vi "SeCrTs-Event logger.vi"(8 "error IO":errorcluster, 11 "?":T1) -> ()   [LabVIEW 2022 SP3]
uses:
  UI Message handler/Message Queue/All Message Queues.ctl
  UI Message handler/Message Queue/Message Cluster.ctl
  Controls/SeCrTs-Control error log.ctl
  UI Message handler/Message Queue/Message Queue.lvlib
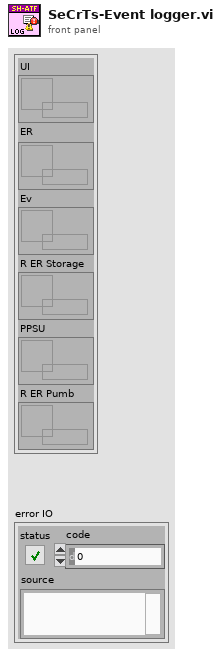
[diagram p1: front panel]
types:
  T1 = typedef "Message Queue.lvlib/All Message Queues.ctl" = cluster{"UI":refnum<queue>, "ER":refnum<queue>, "Ev":refnum<queue>, "R ER Storage":refnum<queue>, "PPSU":refnum<queue>, "R ER Pumb":refnum<queue>}
  T2 = typedef "SeCrTs-Control error log.ctl" = enum16{"Initialise", "Poll Event", "Logg Error", "Exit"}
  T3 = enum16{"open", "replace", "create", "open or create", "replace or create", "replace or create with confirmation"}
  T4 = typedef "SeCrTs-file folder ctl.ctl" = cluster{"Datalog path":path, "Configuration path":path, "Signal list path":path, "Sub vi's":path, "Authentication":path, "Sequence":path, "Event Log":path, "CS Error log":path, "RT Error Log":path}
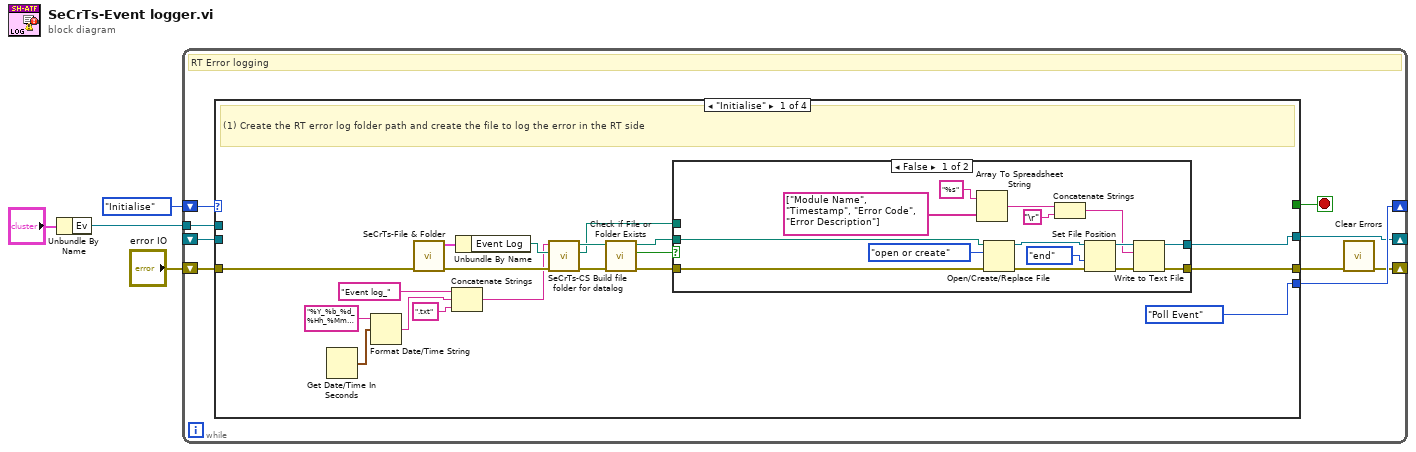
[diagram p0: block diagram]
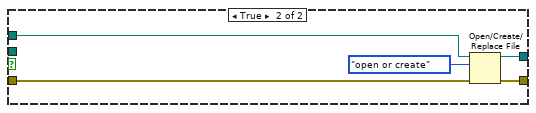
[diagram p2: hidden frame]
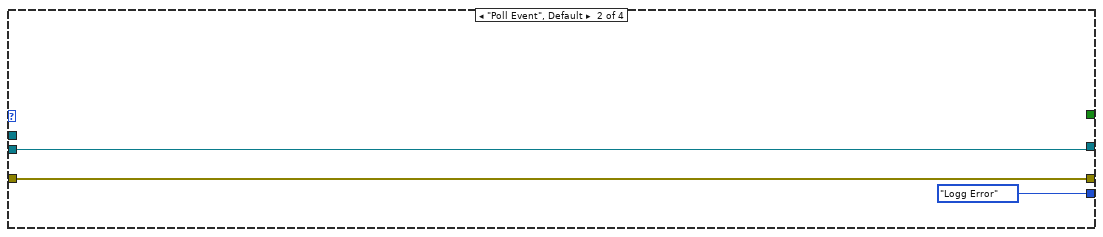
[diagram p3: hidden frame]
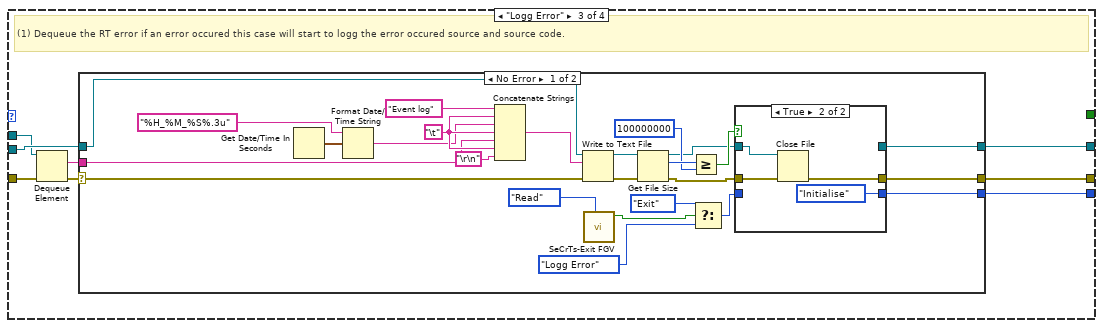
[diagram p4: hidden frame]
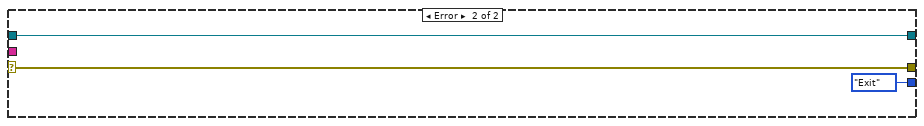
[diagram p6: hidden frame]
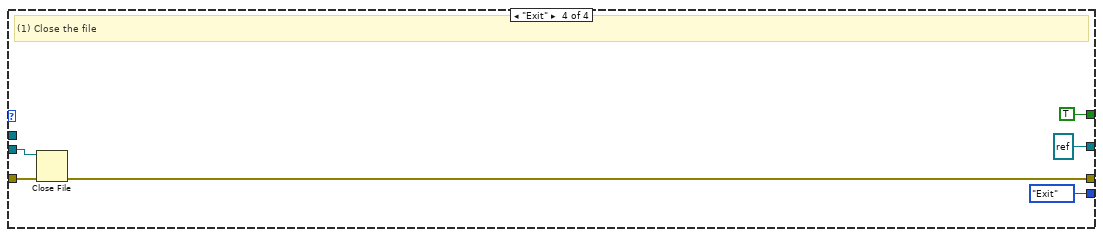
[diagram p7: hidden frame]
diagram:
  n1 = Unbundle By Name("?") -> ("Ev"=w1:refnum<queue>)
  n2 = while {
    shift-right: [w12] -> _
    shift-left: SeCrTs-Control_error_log."Initialise" -> [w13]
    shift-right: [w11] -> _
    shift-left: _ -> [w10]
    shift-right: [w5] -> _
    shift-left: "error IO" -> [w9]
    tunnel: w1 -> [w6]
    stop <- w7 stop-if-true
    # "RT Error logging"
    n3 = case shown="\"Initialise\"" w13 {
      tunnel: [SeCrTs-Control_error_log."Poll Event" SeCrTs-Control_error_log."Logg Error" w57 SeCrTs-Control_error_log."Exit"] -> w12
      tunnel: [w22 w55 w61 refnum<file> refnum ("refnum out")] -> w11
      tunnel: w10 -> [_ w55 w62 w102]
      tunnel: w9 -> [w19 w54 w59 w101]
      tunnel: [w20 w54 w60 w100] -> w8
      tunnel: [_ _ _ TRUE] -> w7
      tunnel: w6 -> [_ _ w56 _]
      frame "Initialise" {
        # "(1) Create the RT error log folder path and create the file to log the error in the RT side"
        n4 = Get Date/Time In Seconds() -> (seconds since 1Jan1904=w15:timestamp)
        n5 = Format Date/Time String(time format string (%c)="%Y_%b_%d_%Hh_%Mm_%Ssec", seconds (now)=w15) -> (date/time string=w14:string)  [unwired: 1 in]
        n6 = call "SeCrTs-File & Folder.vi"("error in (no error)"=w19) -> ("error out"=w31:errorcluster, "File Output"=w32:T4)  [unwired: 9 in]
        n7 = Concatenate Strings("Event log_" ("string"), w14, ".txt" ("string")) -> (w25:string)
        n8 = Unbundle By Name(w32) -> ("Event Log"=w30:path)
        n9 = call "SeCrTs-CS Build file folder for datalog.vi"("error in (no error)"=w31, "Base Path"=w30, "File Name"=w25) -> ("error out"=w28:errorcluster, "Result File path"=w17:path, "Result Folder path"=w29:path)  [unwired: 6 in]
        n10 = call <vilib>:"Check if File or Folder Exists.vi"("error in (no error)"=w28, "path"=w29) -> ("error out"=w21:errorcluster, "file or folder exists?"=w23:bool, "dup path"=w18:path)  [unwired: 7 in]
        n11 = case shown="False" w23 {
          tunnel: [w43 w51] -> w22
          tunnel: w21 -> [w46 w50]
          tunnel: [w42 w49] -> w20
          tunnel: w18 -> [w33 _]
          tunnel: w17 -> [_ w48]
          frame False {
            n12 = Array To Spreadsheet String(array=string[] ["Module Name", "Timestamp", "Error Code", "Error Description"], 3:"%s" ("format string")) -> (spreadsheet string=w37:string)  [unwired: 1 in]
            n13 = Open/Create/Replace File(file path (use dialog)=w33, error in=w46, operation (0:open)=T3."open or create") -> (refnum out=w45:refnum<file>, error out=w44:errorcluster)  [unwired: 3 in, 1 out]
            n14 = Concatenate Strings(w37, "\r") -> (w35:string)
            n15 = Set File Position(refnum=w45, from (0:start)=enum16{"start", "end", "current"}."end", error in=w44) -> (refnum out=w41:refnum<file>, error out=w40:errorcluster)  [unwired: 1 in]
            n16 = Write to Text File(file (use dialog)=w41, text=w35, error in=w40) -> (refnum out=w43:refnum<file>, error out=w42:errorcluster)  [unwired: 1 in, 1 out]
          }
          frame True {
            n17 = Open/Create/Replace File(file path (use dialog)=w48, error in=w50, operation (0:open)=T3."open or create") -> (refnum out=w51:refnum<file>, error out=w49:errorcluster)  [unwired: 3 in, 1 out]
          }
        }
      }
      frame "Poll Event", Default {
      }
      frame "Logg Error" {
        # "(1) Dequeue the RT error if an error occured this case will start to logg the error occured source and source code."
        n18 = Dequeue Element(queue=w56, error in (no error)=w59) -> (element=w63:string, error out=w58:errorcluster)  [unwired: 1 in, 2 out]
        n19 = case shown="No Error" w58 {
          selector: w58 -> [w83 w98]
          tunnel: w63 -> [w66 _]
          tunnel: w62 -> [w88 w97]
          tunnel: [w73 w97] -> w61
          tunnel: [w75 w98] -> w60
          tunnel: [w72 SeCrTs-Control_error_log."Exit"] -> w57
          frame No Error {
            w86 = "\t"
            n20 = Get Date/Time In Seconds() -> (seconds since 1Jan1904=w64:timestamp)
            n21 = Format Date/Time String(time format string (%c)="%H_%M_%S%.3u", seconds (now)=w64) -> (date/time string=w85:string)  [unwired: 1 in]
            n22 = Concatenate Strings("Event log" ("string"), w86, w85, w86, w66, w86, "\r\n") -> (w69:string)
            n23 = Write to Text File(file (use dialog)=w88, text=w69, error in=w83) -> (refnum out=w80:refnum<file>, error out=w81:errorcluster)  [unwired: 1 in, 1 out]
            n24 = call "SeCrTs-Exit FGV.vi"("Enum"=enum16{"Init", "Read", "Write"}."Read") -> ("Exit R"=w68:bool)  [unwired: 9 in, 1 out]
            n25 = Get File Size(file=w80, error in=w81) -> (refnum out=w74:refnum<file>, size (in bytes)=w79:i64, 0:w76:errorcluster)
            n26 = Greater Or Equal?(x=w79, y=i64 100000000) -> (x >= y?=w77:bool)
            n27 = Select(t=SeCrTs-Control_error_log."Exit", s=w68, f=SeCrTs-Control_error_log."Logg Error") -> (s? t:f=w71:T2)
            n28 = case shown="True" w77 {
              tunnel: w76 -> [w91 w93]
              tunnel: [w91 w94] -> w75
              tunnel: w74 -> [w90 w95]
              tunnel: [w90 _] -> w73
              tunnel: [w89 SeCrTs-Control_error_log."Initialise"] -> w72
              tunnel: w71 -> [w89 _]
              frame False {
              }
              frame True {
                n29 = Close File(refnum=w95, error in=w93) -> (error out=w94:errorcluster)  [unwired: 1 out]
              }
            }
          }
          frame Error {
          }
        }
      }
      frame "Exit" {
        # "(1) Close the file"
        n30 = Close File(refnum=w102, error in=w101) -> (error out=w100:errorcluster)  [unwired: 1 out]
      }
    }
    n31 = call <vilib>:"Clear Errors.vi"("error in (no error)"=w8) -> ("error out"=w5:errorcluster)  [unwired: 5 in, 1 out]
  }
